vi "SubVI_GetAtmosphereCorrection.vi"(11 "ErrorIn":errorcluster) -> (1 "bAtmosCorrEnable":bool, 3 "ErrorOut":errorcluster, 4 "u8Error":u8)   [LabVIEW 2013]
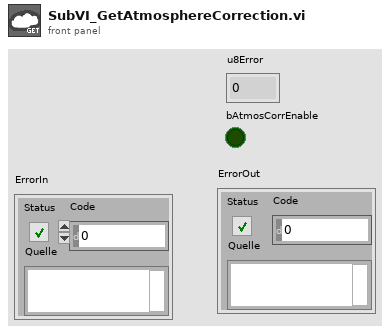
[diagram p1: front panel]
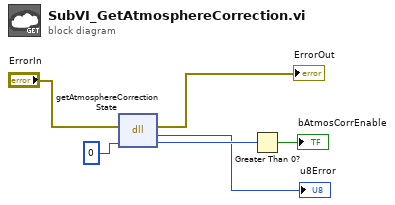
[diagram p0: block diagram]
diagram:
  n1 = dll-call lib="PTH1abs CUsers1000len-bimDesktop&Lieferung_LabView_Interface_11.11.2015Einrichten fÃ¼r - EndkundenDatenTesto_v2013VIlabview_cwrapper_1_0_0.dll" fn="getAtmosphereCorrectionState"(error in="ErrorIn", "u8AtmosCorrState"=u8 0) -> (error out=→"ErrorOut":errorcluster, "u8Error"=→"u8Error":u8, "u8AtmosCorrState"=w2:u8)  [unwired: 2 in, 1 out]
  n2 = Greater Than 0?(x=w2) -> (x > 0?=→"bAtmosCorrEnable":bool)
